vi "worksheet set row opt.vi"(6 "options":cluster{"hidden":u8, "level":u8, "collapsed":u8}, 7 "format":u32, 8 "error in (no error)":errorcluster, 9 "height":dbl, 10 "row":u32, 11 "worksheet":u32) -> (0 "error out":errorcluster, 3 "function return":u32(ring), 4 "options out":cluster{"hidden":u8, "level":u8, "collapsed":u8})   [LabVIEW 2015, in "xlsxwriter.lvlib"]
doc: "lxw_error worksheet_set_row_opt(lxw_worksheet worksheet, lxw_row_t row, double height, lxw_format format, lxw_row_col_options *options);"
uses:
  xlsxwriter.lvlib
  xlsxwriter.dll
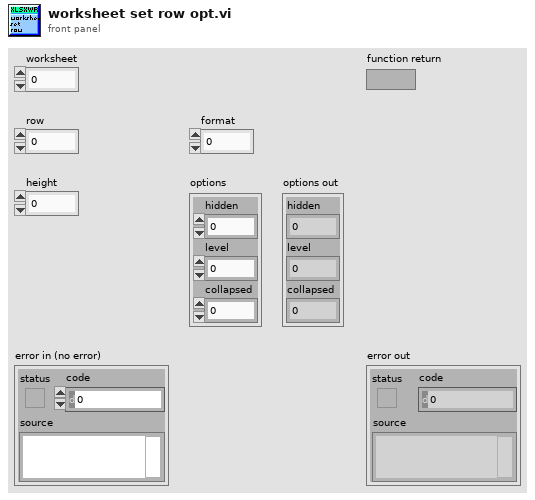
[diagram p1: front panel]
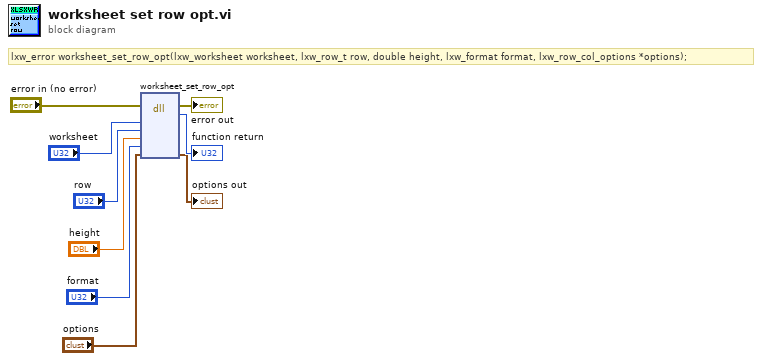
[diagram p0: block diagram]
diagram:
  # "lxw_error worksheet_set_row_opt(lxw_worksheet worksheet, lxw_row_t row, double height, lxw_format format, lxw_row_col_options *options);"
  n1 = dll-call lib="C:/Users/WDAGUtilityAccount/Desktop/lv_vis_added_cell/xlsxwriter.*" fn="worksheet_set_row_opt"(error in="error in (no error)", "worksheet"="worksheet", "row"="row", "height"="height", "format"="format", "options"="options") -> (error out=→"error out":errorcluster, →"function return":u32, "options"=→"options out":cluster{"hidden":u8, "level":u8, "collapsed":u8})  [unwired: 6 in, 1 out]
